vi "ChangeActiveLevels.vi"(6 "Force Update":bool, 8 "Error In":errorcluster, 11 "Active Levels":string[](array[string])) -> (0 "Error Out":errorcluster)   [LabVIEW 2018, in "TracerLibrary.lvlib" / "Tracer.lvclass"]
uses:
  Tracer.lvclass
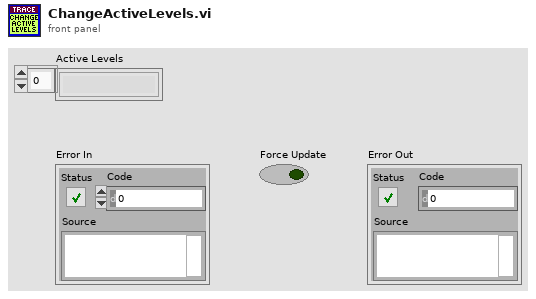
[diagram p1: front panel]
types:
  T1 = typedef "TracerLibrary.lvlib/Tracer.lvclass/TraceItemDefinition.ctl" = cluster{"Item":string, "Enable":bool}
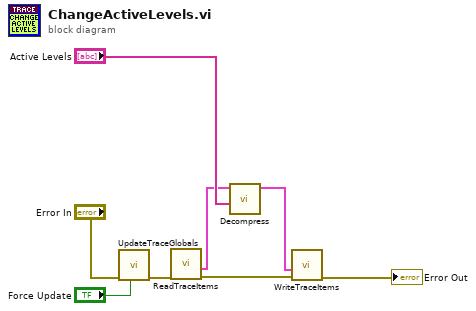
[diagram p0: block diagram]
diagram:
  n1 = call "UpdateTraceGlobals.vi"("Force update"="Force Update", "error in"="Error In") -> ("error out"=w6:errorcluster)  [unwired: 9 in]
  n2 = call "ReadTraceItems.vi"("error in"=w6) -> ("error out"=w7:errorcluster, "TraceItems"=w2:T1[])  [unwired: 9 in]
  n3 = call "Decompress.vi"("Active Compressed in"="Active Levels", "TraceItems in"=w2) -> ("TraceItems out"=w4:cluster{string, bool}[])  [unwired: 9 in]
  n4 = call "WriteTraceItems.vi"("error in"=w7, "TraceItems"=w4) -> ("error out"=→"Error Out":errorcluster)  [unwired: 9 in]
